vi "RG Read (Multiple Waveforms) Splits channels.vi"(8 "error in (no error)":errorcluster, 9 "Maximum Time (10000ms)":u32=10000, 10 "Channels":u16[](array[ring]) items=["Channel 1", "Channel 2", "Channel 3", "Channel 4", "Math", "Reference 1", "Reference 2", "Reference 3", "Reference 4", "D0", "D1", "D2", "D3", "D4", "D5", "D6", "D7", "D8", "D9", "D10", "D11", "D12", "D13", "D14", "D15", "Amplitude", "Frequency", "Phase", "Normal", "Average", "Maximum Peak Hold", "Minimum Peak Hold"], 11 "VISA resource name":refnum<visa-resource-name>) -> (0 "error out":errorcluster, 1 "Channel 2":dynamicdata[](array[waveform]), 2 "Channel 1":dynamicdata[](array[waveform]), 3 "VISA resource name out":refnum<visa-resource-name>)   [LabVIEW 2017, in "Scope.lvlib" / "Tektronix DPO MSO 2000 4000 Series.lvlib"]
doc: "Initiates an acquisition on all channels that you enabled with the <B>Configure Channel</B> VI. The VI waits for the acquisition to complete and returns the waveform for the <B>Channels</B> you specified. The <B>Timeout</B> control specifies the maximum time to wait for operation complete in milliseconds. If the oscilloscope did not complete the acquisition within the time period you specify with the Timeout parameter, the VI returns a timeout error. A common cause for a timeout error is the acquisition was not triggered. For example, the trigger level is out of range of the waveform."
uses:
  Tektronix DPO MSO 2000 4000 Series.lvlib
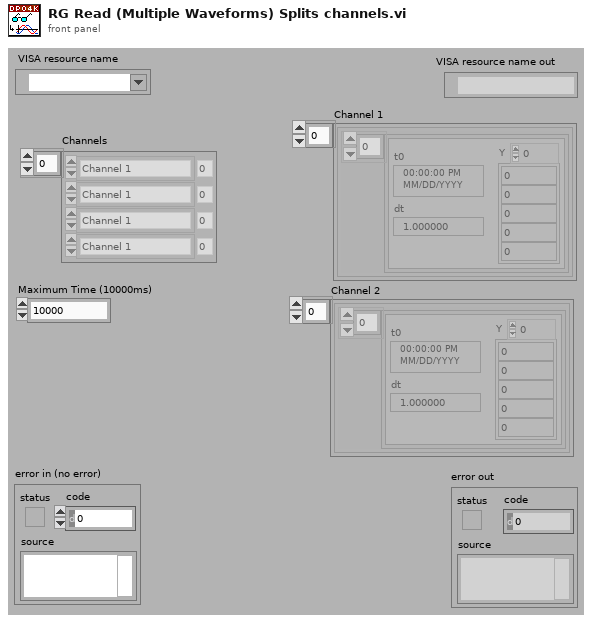
[diagram p1: front panel]
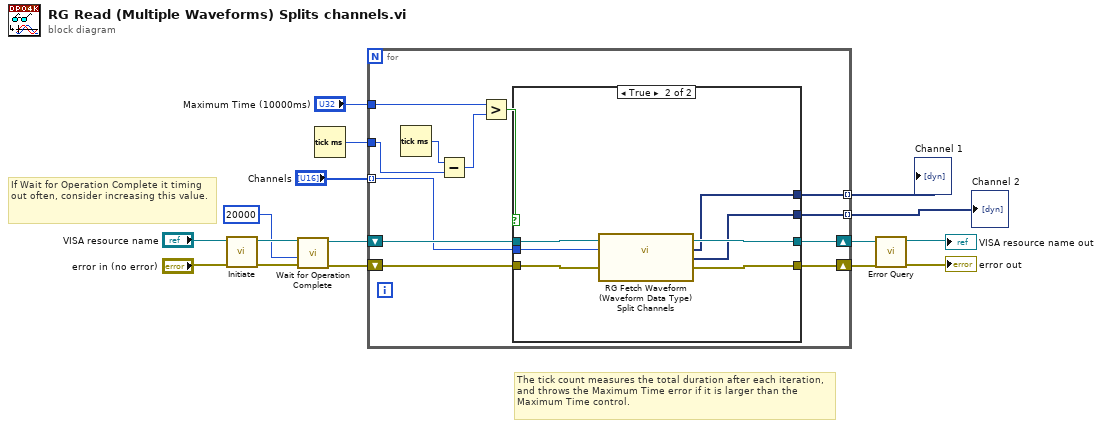
[diagram p0: block diagram]
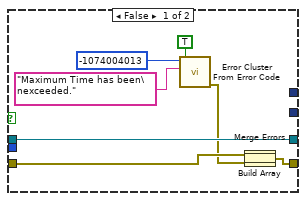
[diagram p2: hidden frame]
diagram:
  # "If Wait for Operation Complete it timing out often, consider increasing this value."
  # "The tick count measures the total duration after each iteration, and throws the Maximum Time error if it is larger than the Maximum Time control."
  n1 = call "Initiate.vi"("error in (no error)"="error in (no error)", "VISA resource name"="VISA resource name") -> ("error out"=w7:errorcluster, "VISA resource name out"=w8:refnum<visa-resource-name>)  [unwired: 8 in]
  n2 = call "Wait for Operation Complete.vi"("error in (no error)"=w7, "Maximum Time (10000ms)"=u32 20000, "VISA resource name"=w8) -> ("error out"=w5:errorcluster, "VISA resource name out"=w6:refnum<visa-resource-name>)  [unwired: 7 in]
  n3 = Tick Count (ms)() -> (millisecond timer value=w3:u32)
  n4 = for {
    shift-right: [w26] -> w15
    shift-left: w6 -> [w27]
    shift-right: [w25] -> w14
    shift-left: w5 -> [w28]
    tunnel: "Channels" -> [w24] mode=indexing
    tunnel: [w23] -> w11 mode=indexing
    tunnel: w3 -> [w21]
    tunnel: "Maximum Time (10000ms)" -> [w20]
    tunnel: [w17] -> w1 mode=indexing
    n5 = Tick Count (ms)() -> (millisecond timer value=w22:u32)
    n6 = Subtract(x=w22, y=w21) -> (x-y=w19:u32)
    n7 = Greater?(x=w20, y=w19) -> (0:w18:bool)
    n8 = case shown="True" w18 {
      tunnel: w28 -> [w31 w43]
      tunnel: w27 -> [w36 w42]
      tunnel: [w36 w41] -> w26
      tunnel: [w32 w40] -> w25
      tunnel: w24 -> [_ w39]
      tunnel: [_ w38] -> w23
      tunnel: [_ w37] -> w17
      frame False {
        n9 = call <vilib>:"Error Cluster From Error Code.vi"("show call chain? (False)"=TRUE, "error message (\"\")"="Maximum Time has been\nexceeded." ("error message (\"\")"), "error code (0)"=-1074004013) -> ("error out"=w30:errorcluster)  [unwired: 6 in]
        n10 = Build Array(w31, w30) -> (w29:errorcluster[])
        n11 = Merge Errors(w29) -> (w32:errorcluster)
      }
      frame True {
        n12 = call "RG Fetch Waveform (Waveform Data Type) Split Channels.vi"("error in (no error)"=w43, "Channel (0: Channel 1)"=w39, "VISA resource name"=w42) -> ("error out"=w40:errorcluster, "Channel 2"=w37:dynamicdata, "Channel 1"=w38:dynamicdata, "VISA resource name out"=w41:refnum<visa-resource-name>)  [unwired: 4 in]
      }
    }
  }
  "Channel 1" <- w11
  "Channel 2" <- w1
  n13 = call "Error Query.vi"("error in (no error)"=w14, "VISA resource name"=w15) -> ("error out"=→"error out":errorcluster, "VISA resource name out"=→"VISA resource name out":refnum<visa-resource-name>)  [unwired: 6 in, 2 out]
